vi "leds.vi"(1 "range (centisec)":dbl, 2 "input":dbl) -> (0 "Output":bool)   [LabVIEW 2011]
uses:
  System Set Points and States.vi
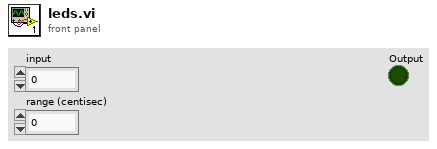
[diagram p1: front panel]
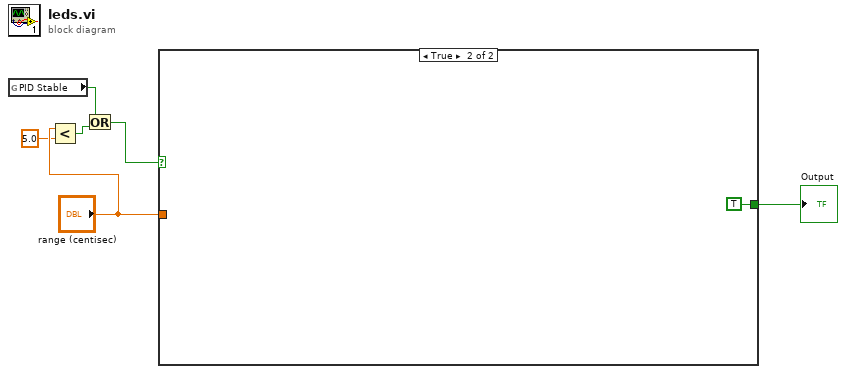
[diagram p0: block diagram]
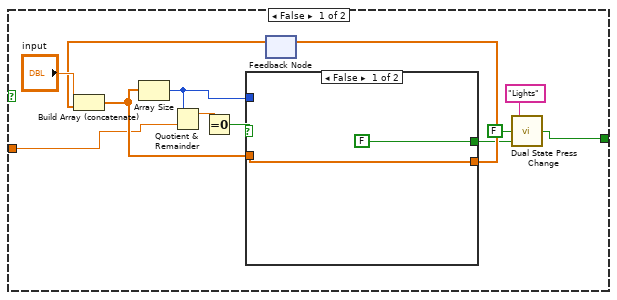
[diagram p2: hidden frame]
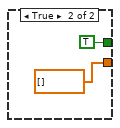
[diagram p3: hidden frame]
diagram:
  n1 = global read "System Set Points and States.vi" "PID Stable"() -> (w1:bool)
  n2 = Less?(x="range (centisec)", y=5.0) -> (x < y?=w3:bool)
  n3 = Or(x=w1, y=w3) -> (x .or. y?=w2:bool)
  n4 = case shown="True" w2 {
    tunnel: "range (centisec)" -> [w11 _]
    tunnel: [w7 TRUE ("Enabled")] -> w4
    frame False {
      n5 = feedback #1() -> (w16:dbl[])  [unwired: 1 in]
      n6 = Build Array (concatenate)("input", w16) -> (w15:dbl[])
      n7 = Array Size(array=w15) -> (size(s)=w14:i32)
      n8 = Quotient & Remainder(x=w14, y=w11) -> (x-y*floor(x/y)=w13:dbl)  [unwired: 1 out]
      n9 = Equal To 0?(x=w13) -> (x = 0?=w12:bool)
      n10 = case shown="False" w12 {
        tunnel: [w20 dbl[] []] -> w17
        tunnel: w15 -> [w20 _]
        tunnel: w14 -> [_ _]
        tunnel: [FALSE TRUE] -> w10
        frame False {
        }
        frame True {
        }
      }
      n11 = feedback-in #1(w17) -> ()
      n12 = call "Dual State Press Change.vi"("Enable/Disable"=w10, "Initial"=FALSE, "Value Name"="Lights") -> ("Enabled"=w7:bool)
    }
    frame True {
    }
  }
  "Output" <- w4
